vi "FTW-Test-JSON-Paths.vi"() -> ()   [LabVIEW 2013]
uses:
  source/Reflection/FTW-Reflection-Type.vi
  source/JSON/FTW-JSON-Core-LibraryFilepath.vi
  source/JSON/FTW-JSON-Core-GetFlattenedValue.vi
  source/JSON/FTW-JSON-Core-LibraryError.vi
  source/CodeGen/JSON Deserialize/FTW-JSON-Deserialize.xnode
panel:
  out "error out":errorcluster
  out "value":cluster{"filepath":string}
  out "Values 2":cluster{"filepath":path}
  out "Values":cluster{"filepath":string}
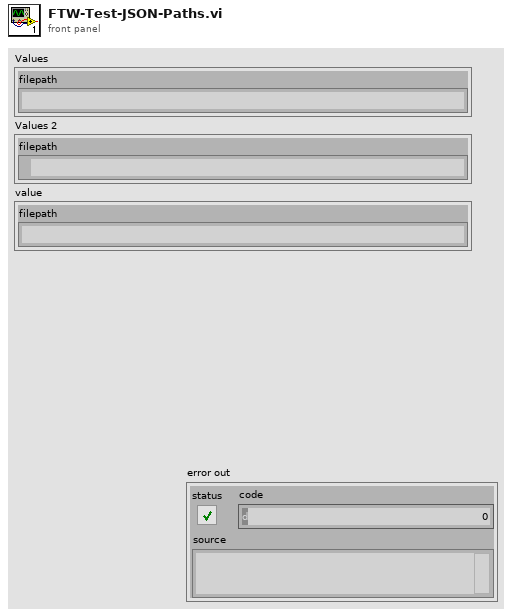
[diagram p1: front panel]
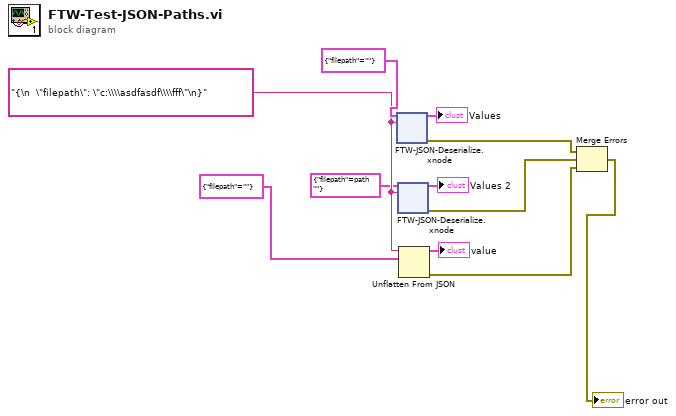
[diagram p0: block diagram]
diagram:
  w9 = "{\n  \"filepath\": \"c:\\\\asdfasdf\\\\fff\"\n}" ("empty string")
  n1 = xnode "FTW-JSON-Deserialize.xnode"("Type and Defaults"=cluster{"filepath":string} {"filepath"=""}, "JSON String"=w9) -> ("Values"=→"Values":cluster{"filepath":string}, "error out"=w4:errorcluster)  [unwired: 1 in]
  n2 = xnode "FTW-JSON-Deserialize.xnode"("Type and Defaults"=cluster{"filepath":path} {"filepath"=path ""}, "JSON String"=w9) -> ("Values"=→"Values 2":cluster{"filepath":path}, "error out"=w3:errorcluster)  [unwired: 1 in]
  n3 = Unflatten From JSON(JSON string=w9, type and defaults=cluster{"filepath":string} {"filepath"=""}) -> (value=→"value":cluster{"filepath":string}, error out=w2:errorcluster)  [unwired: 5 in]
  n4 = Merge Errors(w4, w3, w2) -> (→"error out":errorcluster)
